vi "Spectrometer Triax 550.vi"(7 "Force Reset? (F)":bool, 8 "error in (no error)":errorcluster, 10 "Ref to a Status Box":refnum<vi>, 11 "Spectrometer Triax 550 in":refnum<class "Spectrometer Triax 550.lvclass">) -> (0 "error out":errorcluster, 3 "Spectrometer Triax 550 out":refnum<class "Spectrometer Triax 550.lvclass">)   [LabVIEW 2023, in "Spectrometer Triax 550.lvclass"]
uses:
  Spectrometer Triax 550.lvclass
  Spectrometer Triax 550.lvclass/Spectrometer Triax 550.ctl
  Global/GPIB Numbers.vi
  JY-SPEX-TRIAX/JY-SPEX-TRIAX.lvlib
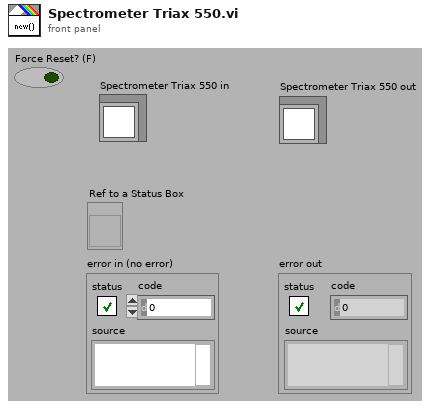
[diagram p1: front panel]
types:
  T1 = typedef "GPIB Type Def.ctl" = cluster{"Name":string, "bus":dbl, "GPIB":dbl, "GPIB as string":string, "byte":i32, "VISA Resource Name":refnum<visa-resource-name>}
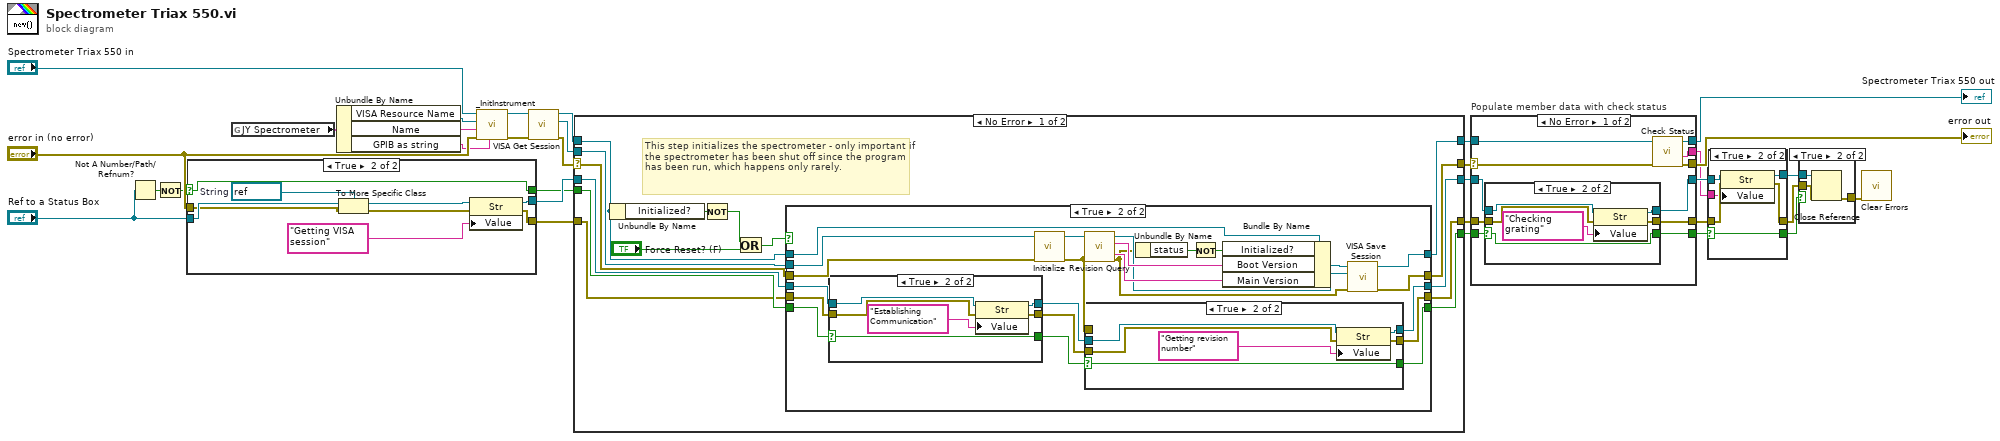
[diagram p0: block diagram]
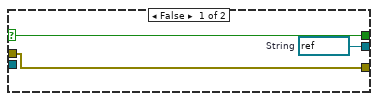
[diagram p4: hidden frame]
diagram:
  n1 = Not A Number/Path/Refnum?(number/path/refnum="Ref to a Status Box") -> (NaN/Path/Refnum?=w16:bool)
  n2 = Not(x=w16) -> (.not. x?=w2:bool)
  n3 = case shown="True" w2 {
    selector: w2 -> [w34 w41]
    tunnel: "error in (no error)" -> [w35 w36]
    tunnel: [w35 w44] -> w25
    tunnel: "Ref to a Status Box" -> [_ w39]
    tunnel: [w33 w42] -> w28
    tunnel: [w34 w41] -> w27
    frame False {
      w33 = refnum<vi> refnum  # String
    }
    frame True {
      w40 = refnum<vi> refnum  # String
      n4 = To More Specific Class(target class=w40, reference=w39, error in=w36) -> (specific class reference=w37:refnum<vi>, error out=w38:errorcluster)
      n5 = property class="Str"(reference=w37, error in=w38, "Value"="Getting VISA session") -> (reference out=w42:refnum<vi>, error out=w44:errorcluster)
    }
  }
  n6 = global read "GPIB Numbers.vi" "JY Spectrometer"() -> (w21:T1)
  n7 = Unbundle By Name(w21) -> ("VISA Resource Name"=w18:refnum<visa-resource-name>, "Name"=w19:string, "GPIB as string"=w20:string)
  n8 = call-dynamic "_InitInstrument.vi"("GPIB as string"=w20, "error in (no error)"="error in (no error)", "Name"=w19, "VISA Resource Name"=w18, "Instrument in"="Spectrometer Triax 550 in") -> ("error out"=w26:errorcluster, "Instrument out"=w15:refnum<class "Spectrometer Triax 550.lvclass">)  [unwired: 1 in, 4 out]
  n9 = call-dynamic "VISA Get Session.vi"("error in (no error)"=w26, "Instrument.lvclass in"=w15) -> ("error out"=w30:errorcluster, "VISA Resource Name"=w31:refnum<visa-resource-name>, "Instrument.lvclass out"=w29:refnum<class "Spectrometer Triax 550.lvclass">)  [unwired: 7 out]
  n10 = case shown="No Error" w30 {
    selector: w30 -> [w50 w110]
    tunnel: [w53 w110] -> w1
    tunnel: w29 -> [w49 w109]
    tunnel: w31 -> [w59 _]
    tunnel: [w58 w109] -> w14
    tunnel: w28 -> [w57 w108]
    tunnel: [w54 w108] -> w11
    tunnel: w27 -> [w56 w107]
    tunnel: [w55 w107] -> w9
    tunnel: w25 -> [w52 w106]
    tunnel: [w51 w106] -> w6
    frame No Error {
      # "This step initializes the spectrometer - only important if the spectrometer has been shut off since the program has been run, which happens only rarely."
      n11 = Unbundle By Name(w49) -> ("Initialized?"=w47:bool)
      n12 = Not(x=w47) -> (.not. x?=w48:bool)
      n13 = Or(x=w48, y="Force Reset? (F)") -> (x .or. y?=w45:bool)
      n14 = case shown="True" w45 {
        tunnel: w49 -> [w64 w83]
        tunnel: w59 -> [_ w82]
        tunnel: [w64 w79] -> w58
        tunnel: w57 -> [w62 w78]
        tunnel: w56 -> [w60 w77]
        tunnel: [w60 w75] -> w55
        tunnel: [w62 w73] -> w54
        tunnel: [w63 w71] -> w53
        tunnel: w52 -> [w61 w70]
        tunnel: [w61 w68] -> w51
        tunnel: w50 -> [w63 w67]
        frame False {
        }
        frame True {
          n15 = case shown="True" w77 {
            selector: w77 -> [w97 w100]
            tunnel: w70 -> [w98 w105]
            tunnel: [w98 w104] -> w69
            tunnel: w78 -> [w99 w103]
            tunnel: [w99 w101] -> w74
            tunnel: [w97 w100] -> w76
            frame False {
            }
            frame True {
              n16 = property class="Str"(reference=w103, error in=w105, "Value"="Establishing Communication") -> (reference out=w101:refnum<vi>, error out=w104:errorcluster)
            }
          }
          n17 = call "Initialize.vi"("error in (no error)"=w67, "VISA resource name"=w82) -> ("error out"=w65:errorcluster, "VISA resource name out"=w87:refnum<visa-resource-name>)  [unwired: 8 out]
          n18 = call "Revision Query.vi"("error in (no error)"=w65, "VISA resource name"=w87) -> ("error out"=w72:errorcluster, "Main Firmware Revision"=w84:string, "Boot Firmware Revision"=w85:string, "VISA resource name out"=w81:refnum<visa-resource-name>)  [unwired: 6 out]
          n19 = case shown="True" w76 {
            selector: w76 -> [w88 w91]
            tunnel: w69 -> [w89 w96]
            tunnel: [w89 w95] -> w68
            tunnel: w74 -> [w90 w94]
            tunnel: [w90 w92] -> w73
            tunnel: [w88 w91] -> w75
            tunnel: w65 -> [_ _]
            frame False {
            }
            frame True {
              n20 = property class="Str"(reference=w94, error in=w96, "Value"="Getting revision number") -> (reference out=w92:refnum<vi>, error out=w95:errorcluster)
            }
          }
          n21 = Unbundle By Name(w72) -> ("status"=w86:bool)
          n22 = Not(x=w86) -> (.not. x?=w66:bool)
          n23 = Bundle By Name(cluster=w83, "Initialized?"=w66, "Boot Version"=w85, "Main Version"=w84) -> (w80:refnum<class "Spectrometer Triax 550.lvclass">)
          n24 = call-dynamic "VISA Save Session.vi"("error in (no error)"=w72, "VISA Resource Name"=w81, "Instrument.lvclass in"=w80) -> ("error out"=w71:errorcluster, "Instrument.lvclass out"=w79:refnum<class "Spectrometer Triax 550.lvclass">)  [unwired: 7 out]
        }
      }
    }
    frame Error {
    }
  }
  n25 = case "Populate member data with check status" shown="No Error" w1 {
    selector: w1 -> [w111 w134]
    tunnel: w14 -> [w121 w135]
    tunnel: [w120 w134] -> w13
    tunnel: [w119 w135] -> w12
    tunnel: w11 -> [w118 w132]
    tunnel: [w117 w132] -> w10
    tunnel: w9 -> [w116 w133]
    tunnel: [w115 w133] -> w8
    tunnel: [w114 w131] -> w7
    tunnel: w6 -> [w113 w131]
    tunnel: [w112 _] -> w5
    frame No Error {
      n26 = case shown="True" w116 {
        selector: w116 -> [w124 w128]
        tunnel: [w122 w130] -> w114
        tunnel: [w124 w128] -> w115
        tunnel: [w123 w127] -> w117
        tunnel: w113 -> [w122 w126]
        tunnel: w118 -> [w123 w125]
        frame False {
        }
        frame True {
          n27 = property class="Str"(reference=w125, error in=w126, "Value"="Checking grating") -> (reference out=w127:refnum<vi>, error out=w130:errorcluster)
        }
      }
      n28 = call-dynamic "Check Status.vi"("error in (no error)"=w111, "Spectrometer Triax 550 in"=w121) -> ("error out"=w120:errorcluster, "Status"=w112:string, "Spectrometer Triax 550 out"=w119:refnum<class "Spectrometer Triax 550.lvclass">)  [unwired: 7 out]
    }
    frame Error {
    }
  }
  "error out" <- w13
  "Spectrometer Triax 550 out" <- w12
  n29 = case shown="True" w8 {
    selector: w8 -> [w138 w142]
    tunnel: [w137 w144] -> w24
    tunnel: [w136 w143] -> w4
    tunnel: [w138 w142] -> w3
    tunnel: w10 -> [w136 w141]
    tunnel: w7 -> [w137 w140]
    tunnel: w5 -> [_ w139]
    frame False {
    }
    frame True {
      n30 = property class="Str"(reference=w141, error in=w140, "Value"=w139) -> (reference out=w143:refnum<vi>, error out=w144:errorcluster)
    }
  }
  n31 = case shown="True" w3 {
    tunnel: w24 -> [w145 w148]
    tunnel: [w145 w147] -> w23
    tunnel: w4 -> [_ w146]
    frame False {
    }
    frame True {
      n32 = Close Reference(reference=w146, error in (no error)=w148) -> (error out=w147:errorcluster)
    }
  }
  n33 = call <vilib>:"Clear Errors.vi"("error in (no error)"=w23) -> ()  [unwired: 1 in, 6 out]
